vi "ParseMessageType.vi"(8 "error in (no error)":errorcluster, 11 "TCP_Server_Connection_Handler in":refnum<class "TCP_Server_Connection_Handler.lvclass">) -> (0 "error out":errorcluster, 3 "TCP_Server_Connection_Handler out":refnum<class "TCP_Server_Connection_Handler.lvclass">)   [LabVIEW 2023, in "TCP_Server_Connection_Handler.lvlib"]
uses:
  TCP_Server_Connection_Handler.lvlib
  TCP_Server_Connection_Handler/TCP_Server_Connection_Handler.lvclass
  TypeDefinitions/messageType.ctl
panel:
  out "message out":string
  out "Filename":string
  out "MessageType":T1
  in  "message in":string
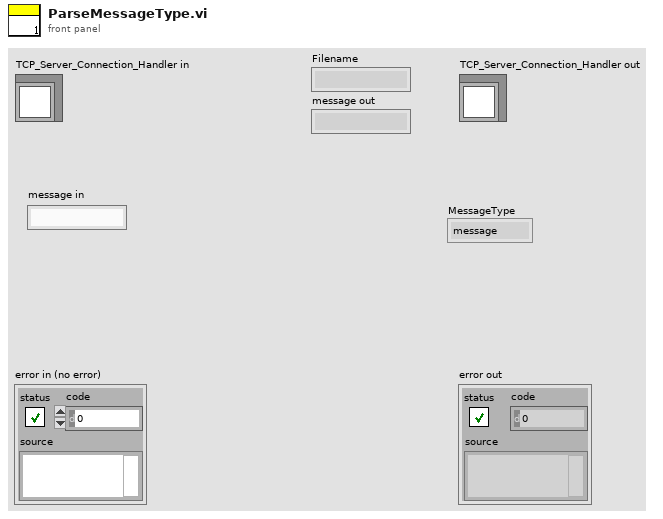
[diagram p1: front panel]
types:
  T1 = typedef "TCP_Server_Connection_Handler.lvlib/messageType.ctl" = enum16{"message", "file", "get"}
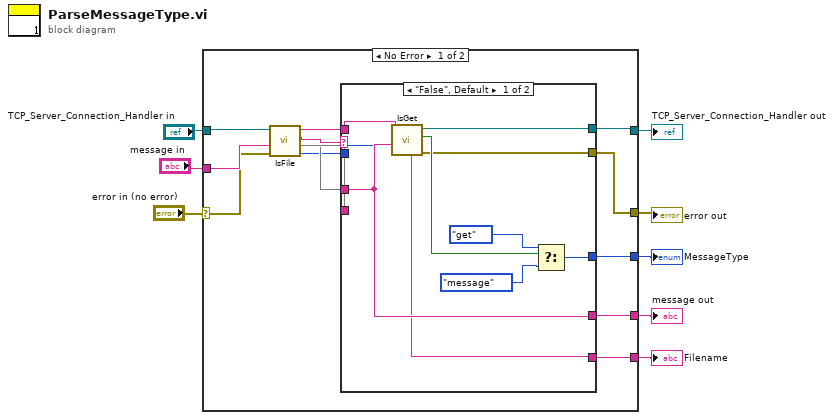
[diagram p0: block diagram]
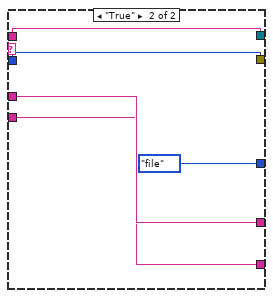
[diagram p2: hidden frame]
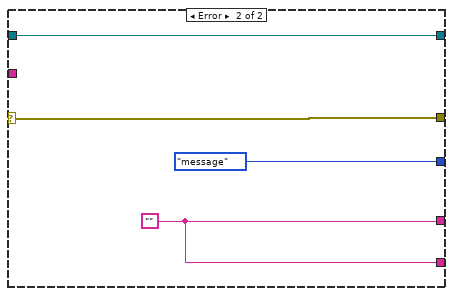
[diagram p3: hidden frame]
diagram:
  n1 = case shown="No Error" "error in (no error)" {
    selector: "error in (no error)" -> [w12 w40]
    tunnel: [w10 w40] -> w7
    tunnel: [w14 w39] -> w5
    tunnel: "TCP_Server_Connection_Handler in" -> [w21 w39]
    tunnel: "message in" -> [w20 _]
    tunnel: [w15 messageType."message" ("MessageType")] -> w3
    tunnel: [w13 w37] -> w2
    tunnel: [w9 w37] -> w1
    frame No Error {
      n2 = call "IsFile.vi"(8:w12, 9:w20, "message in"=w21) -> ("Message type out"=w11:T1, 1:w16, "Filename"=w18:string, "message/data out"=w19:string, 4:w17)  [unwired: 4 in]
      n3 = case shown="\"False\", Default" w18 {
        tunnel: w19 -> [w31 w33]
        tunnel: w17 -> [_ w34]
        tunnel: [w25 messageType."file" ("MessageType")] -> w15
        tunnel: w16 -> [w30 w35]
        tunnel: [w30 w35] -> w9
        tunnel: [w29 w34] -> w13
        tunnel: [w24 w33] -> w14
        tunnel: w11 -> [w23 w32]
        tunnel: [w22 w32] -> w10
        frame "False", Default {
          n4 = call "IsGet.vi"("error in (no error)"=w23, "message in"=w30, "TCP_Server_Connection_Handler in"=w31) -> ("error out"=w22:errorcluster, "IsGet?"=w28:bool, "TCP_Server_Connection_Handler out"=w24:refnum<class "TCP_Server_Connection_Handler.lvclass">, "Filename"=w29:string)  [unwired: 4 in, 1 out]
          n5 = Select(t=messageType."get", s=w28, f=messageType."message" ("MessageType")) -> (s? t:f=w25:T1)
        }
        frame "True" {
        }
      }
    }
    frame Error {
      w37 = ""
    }
  }
  "error out" <- w7
  "TCP_Server_Connection_Handler out" <- w5
  "MessageType" <- w3
  "Filename" <- w2
  "message out" <- w1
